vi "gxml_ReadXMLfromFile.vi"(8 "error in":errorcluster, 11 "XML File Path":path) -> (0 "error out":errorcluster, 2 "XML String Out":string, 3 "XML File Path Out":path)   [LabVIEW 2011, in "Third Party VIs.lvlib" / "GXML.lvlib"]
doc: "This VI opens and reads all data out of an XML file. It strips the file header from the XML string so that the first line of the text string is the opening tag of the first data element."
uses:
  GXML.lvlib
  <vilib>/regexp/Match Regular Expression.xnode
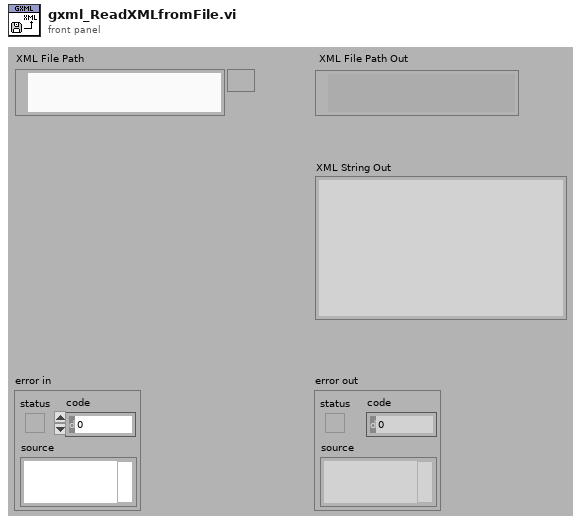
[diagram p1: front panel]
types:
  T1 = enum16{"open", "replace", "create", "open or create", "replace or create", "replace or create with confirmation"}
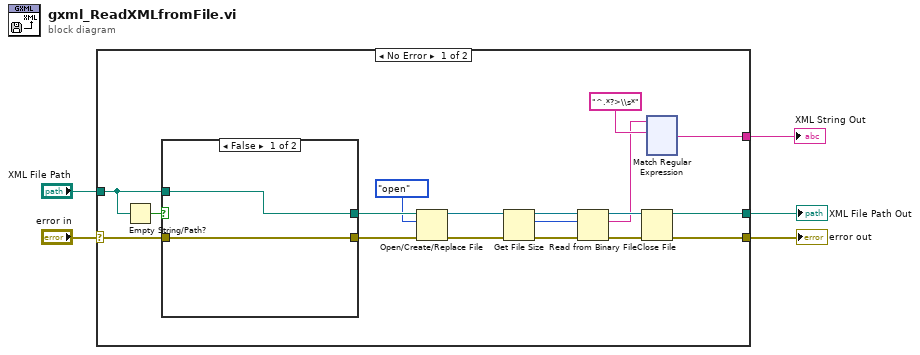
[diagram p0: block diagram]
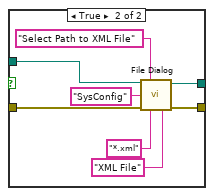
[diagram p2: hidden frame]
diagram:
  n1 = case shown="No Error" "error in" {
    selector: "error in" -> [w20 w147]
    tunnel: [w15 w147] -> w4
    tunnel: [w23 w146] -> w3
    tunnel: "XML File Path" -> [w19 w146]
    tunnel: [w12 ""] -> w1
    frame No Error {
      n2 = Empty String/Path?(string/path=w19) -> (empty?=w18:bool)
      n3 = case shown="False" w18 {
        tunnel: w20 -> [w136 w144]
        tunnel: [w135 w139] -> w16
        tunnel: [w136 w138] -> w17
        tunnel: w19 -> [w135 w137]
        frame False {
        }
        frame True {
          n4 = call "File Dialog"("start path"=w137, "prompt"="Select Path to XML File" ("Prompt"), "default name"="SysConfig", "error in"=w144, "pattern (all files)"="*.xml" ("pattern"), "pattern label"="XML File") -> ("selected path"=w139:path, "error out"=w138:errorcluster)  [unwired: 6 in, 2 out]
        }
      }
      n5 = Open/Create/Replace File(file path (use dialog)=w16, error in=w17, operation (0:open)=T1."open") -> (refnum out=w8:refnum<file>, error out=w10:errorcluster)  [unwired: 3 in, 1 out]
      n6 = Get File Size(file=w8, error in=w10) -> (refnum out=w7:refnum<file>, size (in bytes)=w6:i64, 0:w9:errorcluster)
      n7 = Read from Binary File(8:w9, 10:w6, 11:w7) -> (0:w21:errorcluster, 2:w11:string, 3:w22:refnum<file>)  [unwired: 3 in, 1 out]
      n8 = Close File(refnum=w22, error in=w21) -> (path=w23:path, error out=w15:errorcluster)
      n9 = xnode "Match Regular Expression"("input string"=w11, "regular expression"="^.*?>\\s*") -> ("after match"=w12:string)  [unwired: 4 in, 4 out]
    }
    frame Error {
    }
  }
  "error out" <- w4
  "XML File Path Out" <- w3
  "XML String Out" <- w1
